vi "GEN_Plain_track_overlay_PIC.vi"(7 "Image size":cluster{"x":i32, "y":i32}={"x"=480, "y"=480}, 8 "Error In":errorcluster, 9 "Samples full merge, every N":i32=10000, 10 "Multiline grouping, samples":i32=100, 11 "Full track array":T1(array[cluster])) -> (0 "Error Out":errorcluster, 3 "Plain track overlay pixmap":u32[][](array[numeric]) format="%x")   [LabVIEW 2018, in "Tracker.lvlib"]
uses:
  Tracker.lvlib
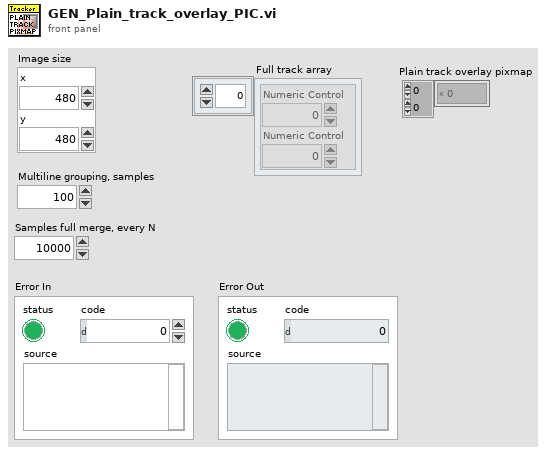
[diagram p1: front panel]
types:
  T1 = cluster{"Numeric Control":dbl, "Numeric Control":dbl}[]
  T2 = cluster{"Left":i32, "Top":i32, "Right":i32, "Bottom":i32}
  T3 = cluster{"Width":i16, "Style":enum32{"Solid", "Dash", "Dot", "DashDot", "DashDotDot"}}
  T4 = cluster{"Numeric Control":dbl, "Numeric Control":dbl}
  T5 = cluster{"Width":u16, "Style":enum32{"Solid", "Dash", "Dot", "DashDot", "DashDotDot"}}
  T6 = typedef "imagedata.ctl" = cluster{"image type":i32, "image depth":i32, "image":u8[], "mask":u8[], "colors":u32[], "Rectangle":cluster{"left":i16, "top":i16, "right":i16, "bottom":i16}}
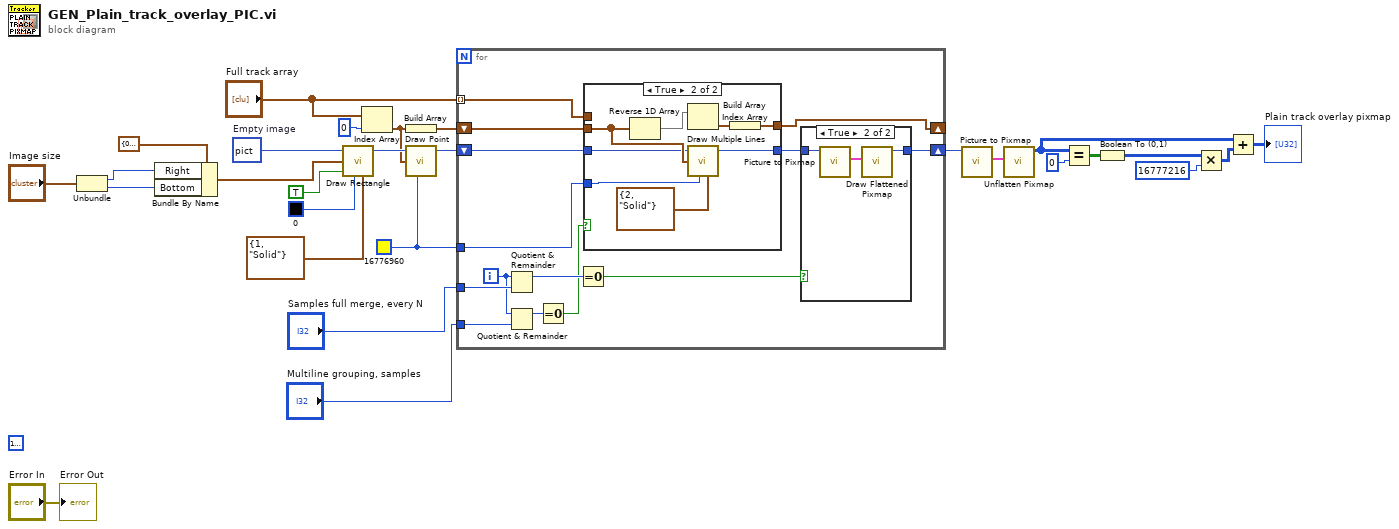
[diagram p0: block diagram]
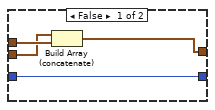
[diagram p2: hidden frame]
diagram:
  w1 = u32 16776960 ("color(black)")
  (unwired) u32 16777216
  w14 = picture data[5B]  # Empty image
  n1 = Unbundle("Image size") -> ("x"=w26:i32, "y"=w27:i32)
  n2 = Bundle By Name(cluster=T2 {"Left"=0, "Top"=0, "Right"=0, "Bottom"=0} ("Rectangle"), "Right"=w26, "Bottom"=w27) -> (w28:T2)
  n3 = call <vilib>:"Draw Rectangle.vi"("picture"=w14, "rect"=w28, "fill?(F)"=TRUE, "color(black)"=u32 0, "pen"=T3 {"Width"=1, "Style"=enum."Solid"}) -> ("new picture"=w23:picture)  [unwired: 4 in]
  n4 = Index Array(array="Full track array", index=0) -> (element=w18:T4)
  n5 = Build Array(w18) -> (w19:T1)
  n6 = call <vilib>:"Draw Point.vi"("picture"=w23, "point(x,y)"=w18, "color(black)"=w1) -> ("new picture"=w17:picture)  [unwired: 6 in]
  n7 = for {
    shift-right: [w39] -> w20
    shift-left: w17 -> [w38]
    tunnel: "Full track array" -> [w33] mode=indexing
    tunnel: "Samples full merge, every N" -> [w40]
    tunnel: "Multiline grouping, samples" -> [w35]
    shift-right: [w31] -> _
    shift-left: w19 -> [w32]
    tunnel: w1 -> [w29]
    i -> [w36]
    n8 = Quotient & Remainder(x=w36, y=w40) -> (x-y*floor(x/y)=w41:i32)  [unwired: 1 out]
    n9 = Quotient & Remainder(x=w36, y=w35) -> (x-y*floor(x/y)=w37:i32)  [unwired: 1 out]
    n10 = Equal To 0?(x=w37) -> (x = 0?=w30:bool)
    n11 = Equal To 0?(x=w41) -> (x = 0?=w42:bool)
    n12 = case shown="True" w30 {
      tunnel: w38 -> [w46 w50]
      tunnel: [w46 w49] -> w34
      tunnel: w33 -> [w45 _]
      tunnel: w32 -> [w44 w51]
      tunnel: [w43 w48] -> w31
      tunnel: w29 -> [_ w47]
      frame False {
        n13 = Build Array (concatenate)(w44, w45) -> (w43:T1)
      }
      frame True {
        n14 = Reverse 1D Array(array=w51) -> (reversed array=w54:T1)
        n15 = Index Array(array=w54) -> (element=w53:T4)  [unwired: 1 in]
        n16 = call <vilib>:"Draw Multiple Lines.vi"("picture"=w50, "line endpoints"=w51, "color(black)"=w47, "pen"=T5 {"Width"=2, "Style"=enum."Solid"}) -> ("new picture"=w49:picture)  [unwired: 5 in]
        n17 = Build Array(w53) -> (w48:T1)
      }
    }
    n18 = case shown="True" w42 {
      tunnel: [w55 w57] -> w39
      tunnel: w34 -> [w55 w56]
      frame False {
      }
      frame True {
        n19 = call <vilib>:"Picture to Pixmap.vi"("picture"=w56) -> ("image data"=w58:T6)  [unwired: 9 in, 1 out]
        n20 = call <vilib>:"Draw Flattened Pixmap.vi"("image data"=w58) -> ("new picture"=w57:picture)  [unwired: 8 in]
      }
    }
  }
  n21 = call <vilib>:"Picture to Pixmap.vi"("picture"=w20) -> ("image data"=w11:T6)  [unwired: 9 in, 1 out]
  n22 = call <vilib>:"Unflatten Pixmap.vi"("image data"=w11) -> ("24-bit pixmap"=w3:u32[][])  [unwired: 4 in, 6 out]
  n23 = Equal?(x=w3, y=0) -> (x = y?=w7:bool[][])
  n24 = Boolean To (0,1)(Boolean=w7) -> (0, 1=w6:i16[][])
  n25 = Multiply(x=w6, y=16777216) -> (x*y=w4:i32[][])
  n26 = Add(x=w3, y=w4) -> (x+y=→"Plain track overlay pixmap":u32[][])
  "Error Out" <- "Error In"
